vi "Toggle Field Panel.vi"(8 "error in (no error)":errorcluster, 11 "SB App in":refnum<class "SB App.lvclass">) -> (0 "error out":errorcluster, 3 "SB App out":refnum<class "SB App.lvclass">)   [LabVIEW 2020, in "SB App.lvlib" / "SB App.lvclass"]
uses:
  SB App.lvclass
  SB App.lvclass/SB App.ctl
  Team Field Panel/Team Field Panel.lvclass
  C:/Program Files (x86)/National Instruments/LabVIEW 2020/vi.lib/IlluminatedG/IG OOPanel/OOPanel/Panel/Panel.lvclass
  Square Field Panel/Square Field Panel.lvclass
  <vilib>/IlluminatedG/IG OOPanel/OOPanel/Manager/Manager.lvclass
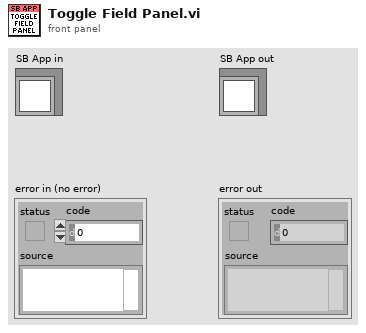
[diagram p1: front panel]
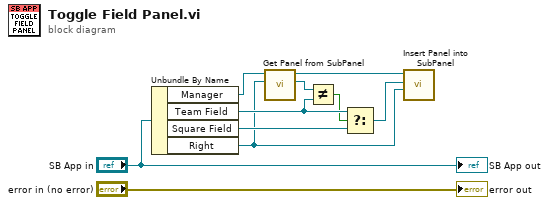
[diagram p0: block diagram]
diagram:
  n1 = Unbundle By Name("SB App in") -> ("Manager"=w8:refnum<class "Manager.lvclass">, "Team Field"=w6:refnum<class "Team Field Panel.lvclass">, "Square Field"=w5:refnum<class "Square Field Panel.lvclass">, "Right"=w1:refnum<vi>)
  n2 = call <vilib>:"Get Panel from SubPanel.vi"("SubPanel"=w1, "Manager in"=w8) -> ("Panel"=w7:refnum<class "Panel.lvclass">, "Manager out"=w3:refnum<class "Manager.lvclass">)  [unwired: 7 in, 1 out]
  n3 = Not Equal?(x=w7, y=w6) -> (x != y?=w4:bool)
  n4 = Select(t=w6, s=w4, f=w5) -> (s? t:f=w2:refnum<class "Panel.lvclass">)
  n5 = call <vilib>:"Insert Panel into SubPanel.vi"("SubPanel"=w1, "Panel In"=w2, "Manager in"=w3) -> ()  [unwired: 6 in, 3 out]
  "error out" <- "error in (no error)"
  "SB App out" <- "SB App in"
